vi "Connections to Strings.vi"(11 "connection list":T1[](array[typedef])) -> (3 "connection strings":string[](array[string]))   [LabVIEW 2017, in "SLSC Switch Scripting.lvlib"]
uses:
  SLSC Switch Scripting.lvlib
  Routing Channel/Connection.ctl
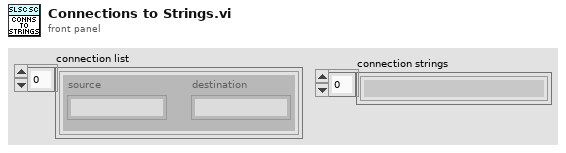
[diagram p1: front panel]
types:
  T1 = typedef "SLSC Switch Scripting.lvlib/Connection.ctl" = cluster{"source":string, "destination":string}
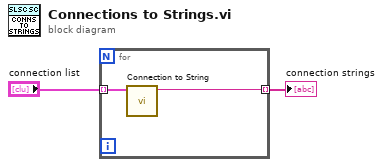
[diagram p0: block diagram]
diagram:
  n1 = for {
    tunnel: "connection list" -> [w4] mode=indexing
    tunnel: [w3] -> w1 mode=indexing
    n2 = call "Connection to String.vi"("Connection"=w4) -> ("String"=w3:string)  [unwired: 10 in]
  }
  "connection strings" <- w1
